vi "HFRR ADV v02.vi"() -> ()   [LabVIEW 2023] (continued)
    n419 = local read "EXIT"() -> (w418:bool)
    "Error Uno" <- w412
  }
  n420 = while {
    tunnel: w47 -> [_]
    tunnel: [w801] -> _
    tunnel: w16 -> [_]
    tunnel: ["EXIT"] -> w44
    i -> [w801]
    stop <- "EXIT" stop-if-true
    # "C:\\LAB-IQ-NXT\\Scar View.exe"
    n421 = local read "RUN"() -> (w799:bool)
    n422 = local read "EDIT 2"() -> (w786:bool)
    n423 = case shown="False" w799 {
      frame False {
        n424 = local read "stopT"() -> (w1691:bool)
        n425 = case shown="True" w1691 {
          frame False {
          }
          frame True {
            w1692 = FALSE
            n426 = local write "st enable"(w1692) -> ()
            n427 = local write "stopT"(w1692) -> ()
          }
        }
      }
      frame True {
        "stopT" <- TRUE
      }
    }
    n428 = case shown="True" w786 {
      frame False {
        n429 = local write "Password 2"("" ("Password")) -> ()
        n430 = property on="Password 2" class="Str"("Visible"=FALSE) -> ()  [unwired: 2 in, 2 out]
      }
      frame True {
        n431 = property on="Password 2" class="Str"("Visible"=TRUE) -> ()  [unwired: 2 in, 2 out]
        n432 = Equal?(x="Password 2", y="HFRR1234") -> (x = y?=w831:bool)
        n433 = case shown="True" w831 {
          tunnel: "Password 2" -> [w834 _]
          frame False {
            n434 = String Length(string=w834) -> (length=w835:i32)
            n435 = Greater Than 0?(x=w835) -> (x > 0?=w833:bool)
            n436 = case shown="False" w833 {
              frame False {
                n437 = property on="Password 2" class="Str"("Caption.Text"="Password (Advance Setting)") -> ()  [unwired: 2 in, 2 out]
              }
              frame True {
                n438 = property on="Password 2" class="Str"("Caption.Text"="Incorrect Password!") -> ()  [unwired: 2 in, 2 out]
              }
            }
          }
          frame True {
            n439 = local write "Password 2"("" ("Password")) -> ()
            n440 = local write "Main Tab"(T1."Advance" ("Main Tab")) -> ()
            n441 = local write "EDIT 2"(FALSE ("EDIT 2")) -> ()
          }
        }
      }
    }
    n442 = Wait (ms)(milliseconds to wait=u32 50) -> ()  [unwired: 1 out]
    n443 = local read "EXIT 2"() -> (w779:bool)
    n444 = local read "Configure"() -> (w782:bool)
    n445 = local read "Analysis"() -> (w781:bool)
    n446 = local read "Home 9"() -> (w776:bool)
    n447 = local read "Home"() -> (w775:bool)
    n448 = local read "STOP 2"() -> (w778:bool)
    n449 = local read "Home 8"() -> (w777:bool)
    n450 = case shown="True" "EDIT 3" {
      frame False {
      }
      frame True {
        n451 = local write "EDIT 3"(FALSE ("EDIT 3")) -> ()
        n452 = local write "Main Tab"(T1."About" ("Main Tab")) -> ()
      }
    }
    n453 = local read "Re-Initialise"() -> (w784:bool)
    n454 = case shown="True" w779 {
      selector: w779 -> [_ w812]
      frame False {
      }
      frame True {
        n455 = local write "EXIT"(w812) -> ()
        n456 = local write "EXIT 2"(FALSE ("EXIT 2")) -> ()
        n457 = local write "Main Tab"(T1."HOME" ("Main Tab")) -> ()
      }
    }
    n458 = case shown="True" w775 {
      frame False {
      }
      frame True {
        (unwired) T10."HOME" ("Main Tab")
        n459 = local write "Home"(FALSE ("Home")) -> ()
        n460 = local write "Main Tab"(T1."HOME" ("Main Tab")) -> ()
      }
    }
    n461 = case shown="True" w784 {
      frame False {
      }
      frame True {
        n462 = local write "Re-Initialise"(FALSE ("Re-Initialise")) -> ()
      }
    }
    n463 = case shown="True" w776 {
      frame False {
      }
      frame True {
        n464 = local write "Main Tab"(T1."HOME" ("Main Tab")) -> ()
        n465 = local write "Home 9"(FALSE ("Home 9")) -> ()
      }
    }
    n466 = case shown="True" w777 {
      frame False {
      }
      frame True {
        n467 = local write "Home 8"(FALSE ("Home 8")) -> ()
        n468 = local write "Main Tab"(T1."HOME" ("Main Tab")) -> ()
      }
    }
    n469 = case shown="True" w778 {
      frame False {
      }
      frame True {
        n470 = local write "STOP 2"(FALSE ("STOP 2")) -> ()
        n471 = local write "Main Tab"(T1."HOME" ("Main Tab")) -> ()
      }
    }
    n472 = case shown="True" w782 {
      frame False {
      }
      frame True {
        n473 = local write "Configure"(FALSE) -> ()
        n474 = local write "Main Tab"(T1."Acquire" ("Main Tab")) -> ()
      }
    }
    n475 = local read "service 2"() -> (w780:bool)
    n476 = case shown="True" w781 {
      frame False {
      }
      frame True {
        n477 = local write "Analysis"(FALSE) -> ()
        n478 = local write "Main Tab"(T1."Compare Files" ("Main Tab")) -> ()
      }
    }
    n479 = case shown="\"ASTM D6079\", Default" "TEST STANDARD" {
      tunnel: [2.0 ("Set Temp") 0.0 ("Set Temp") 2.0 ("Set Temp") 0.0 ("Set Temp")] -> w787
      frame "ASTM D6079", Default {
        # "astm hide"
        n480 = local write "Set Hz"(50.0 ("Hz")) -> ()
        n481 = local write "Set Strk"(1.0 ("Set Strk")) -> ()
        n482 = local write "Set Rh"(53.0 ("Set Rh")) -> ()
        n483 = local write "Set Temp"(60.0 ("Set Temp")) -> ()
        n484 = local write "test time"(75.0 ("test time")) -> ()
        n485 = local write "NORMAL LOAD"(2.0 ("NORMAL LOAD")) -> ()
        "Test Standard" <- "ASTM D6079" ("Test Standard 2")
      }
      frame "ISO 12156" {
        n486 = local write "Set Hz"(50.0 ("Hz")) -> ()
        n487 = local write "Set Rh"(53.0 ("Set Rh")) -> ()
        n488 = local write "Set Strk"(1.0 ("Set Strk")) -> ()
        n489 = local write "test time"(75.0 ("test time")) -> ()
        n490 = local write "Set Temp"(60.0 ("Set Temp")) -> ()
        n491 = local write "NORMAL LOAD"(2.0 ("NORMAL LOAD")) -> ()
      }
      frame "CEC F-096-A-06" {
        n492 = local write "Set Strk"(1.0 ("Set Strk")) -> ()
        n493 = local write "Set Hz"(50.0 ("Hz")) -> ()
        n494 = local write "Set Rh"(53.0 ("Set Rh")) -> ()
        n495 = local write "Set Temp"(60.0 ("Set Temp")) -> ()
        n496 = local write "test time"(75.0 ("test time")) -> ()
        n497 = local write "NORMAL LOAD"(2.0 ("NORMAL LOAD")) -> ()
      }
      frame "Custom" {
      }
    }
    n498 = local read "OPEN 6"() -> (w783:bool)
    n499 = local read "service 3"() -> (w773:bool)
    n500 = case shown="True" w780 {
      frame False {
      }
      frame True {
        n501 = local write "service 2"(FALSE) -> ()
        n502 = local write "Main Tab"(T1."About" ("Main Tab")) -> ()
      }
    }
    n503 = Or(x=w783, y=w773) -> (x .or. y?=w774:bool)
    n504 = local read "RUN"() -> (w796:bool)
    n505 = case shown="True" w774 {
      selector: w774 -> [_ w823]
      frame False {
      }
      frame True {
        n506 = Not(x=w823) -> (.not. x?=w819:bool)
        n507 = local write "service 3"(w819) -> ()
        n508 = local write "OPEN 6"(w819) -> ()
        n509 = call <vilib>:"System Exec.vi"("wait until completion? (T)"=TRUE, "command line"="C:\\LAB-IQ-NXT\\Scar View.exe") -> ("error out"=→"error out 5":errorcluster)  [unwired: 6 in, 3 out]
      }
    }
    n510 = case shown="True" w796 {
      frame False {
      }
      frame True {
        n511 = local read "Main Tab"() -> (w1689:T1)
        n512 = case shown="\"Compare Files\"" w1689 {
          frame "Acquire", Default {
          }
          frame "Compare Files" {
            n513 = local write "Main Tab"(T1."Acquire" ("Main Tab")) -> ()
          }
          frame "About" {
          }
        }
      }
    }
    n514 = local read "Main Tab"() -> (w772:T1)
    n515 = case shown="\"Compare Files\"" w772 {
      tunnel: [T10."Acquire" ("Main Tab") T11."   COMPARE   FILES " ("Tab Control") T12."PRINT REPORT" ("Tab Control")] -> w794
      frame "Acquire", Default {
      }
      frame "Compare Files" {
      }
      frame "About" {
      }
    }
    n516 = property on="SetTemp" class="DigNum (strict)"("Disabled"=w787) -> ()  [unwired: 2 in, 2 out]
    n517 = case shown="0, Default" w794 {
      frame 0, Default {
        w1833 = 0.2 ("y")
        w1838 = 1.0 ("y")
        w1839 = 0.8 ("y")
        # "Elapsed time\ncof\nstroke\nAir temp\nTemp\nHumidity"
        n518 = case shown="True" "Save & Continue" {
          frame False {
          }
          frame True {
            "acq 2" <- TRUE ("acq 2")
          }
        }
        n519 = case shown="True" "Save & Continue" {
          frame False {
          }
          frame True {
            n520 = while {
              tunnel: "0123456789abcdefghijklmnopqrstuvwxyzABCDEFGHIJKLMNOPQRSTUVWXYZ" ("string 2") -> [w1957]
              shift-right: [w1955] -> w1950
              shift-left: "" -> [w1954]
              i -> [w1964]
              stop <- w1963 stop-if-true
              n521 = Random Number (0-1)() -> (number: 0 to 1=w1958:dbl)
              n522 = Multiply(x=w1958, y=62.0) -> (x*y=w1960:dbl)
              n523 = Decrement(x="Length") -> (x-1=w1953:i16)
              n524 = To Word Integer(number=w1960) -> (16bit integer=w1961:i16)
              n525 = String Subset(string=w1957, offset (0)=w1961, length (rest)=1 ("length (rest)")) -> (substring=w1956:string)
              n526 = Greater Or Equal?(x=w1964, y=w1953) -> (x >= y?=w1963:bool)
              n527 = Concatenate Strings(w1956, w1954) -> (w1955:string)
            }
            n528 = local write "UUID"(w1950) -> ()
          }
        }
        n529 = case shown="True" "Save & Continue" {
          frame False {
          }
          frame True {
            n530 = local read "Operator ID"() -> (w2240:string)
            n531 = local read "FILE"() -> (w2247:string)
            n532 = String Length(string=w2240) -> (length=w2241:i32)
            n533 = String Length(string=w2247) -> (length=w2245:i32)
            n534 = Greater?(x=w2241, y=0) -> (0:w2239:bool)
            n535 = Greater?(x=w2245, y=0) -> (0:w2244:bool)
            n536 = And(x=w2244, y=w2239) -> (x .and. y?=w2243:bool)
            n537 = case shown="True" w2243 {
              frame False {
                n538 = stacked-sequence {
                  frame #0 {
                    n539 = One Button Dialog(message="Please Enter a File Name and Operator ID to save data !", button name ("OK")="Ok") -> ()  [unwired: 1 out]
                  }
                  frame #1 {
                    n540 = local write "Save & Continue"(FALSE ("OK Button")) -> ()
                  }
                }
                n541 = local write "Save & Continue"(FALSE ("OK Button")) -> ()
              }
              frame True {
                n542 = stacked-sequence {
                  frame #0 {
                    (unwired) ")!" ("string")
                    (unwired) ")" ("string")
                    w2252 = dbl[] [] ("History Data")
                    w2256 = "\r"
                    # "C:\\WinDucom\\Data\\"
                    # "C:\\LAB-IQ-NXT\\data"
                    n543 = local read "Batch Ref Num :"() -> (w2254:string)
                    n544 = local read "NORMAL LOAD"() -> (w2273:dbl)
                    n545 = local read "Fuel Discription :"() -> (w2267:string)
                    n546 = Multiply(x=w2273, y=1.0) -> (x*y=w2272:dbl)
                    n547 = Number To Fractional String(number=w2272, width (-)=i16 5, precision (6)=i16 2) -> (F-format string=w2281:string)  [unwired: 1 in]
                    n548 = Concatenate Strings(w2267) -> (w2268:string)
                    n549 = local read "Remarks :"() -> (w2266:string)
                    n550 = property on="Electronic contact resistance ( % )" class="WFChart (strict)"("History Data"=w2252) -> ()  [unwired: 2 in, 2 out]
                    n551 = Get Date/Time String(date format (0)=enum16{"short", "long", "abbreviated"}."short") -> (date string=w2292:string, time string=w2289:string)  [unwired: 2 in]
                    n552 = property on="Coefficient of Friction" class="WFChart (strict)"("History Data"=w2252) -> ()  [unwired: 2 in, 2 out]
                    n553 = property on="Frictional Force ( N )" class="WFChart (strict)"("History Data"=w2252) -> ()  [unwired: 2 in, 2 out]
                    n554 = Concatenate Strings(w2254) -> (w2253:string)
                    n555 = Concatenate Strings(w2266, "," ("string")) -> (w2265:string)
                    n556 = Concatenate Strings("Load :- " ("Substring"), w2281, " N ," ("Substring")) -> (w2280:string)
                    n557 = local read "String 41"() -> (w2258:string)
                    n558 = local read "FILE"() -> (w2300:string)
                    n559 = Concatenate Strings("(" ("Substring"), w2292, ")" ("Substring"), w2289) -> (w2260:string)
                    "concatenated string" <- w2260
                    n560 = Concatenate Strings("C:\\LAB-IQ-NXT\\data\\" ("string"), w2300) -> (w2299:string)
                    n561 = Concatenate Strings("tested by") -> (w2262:string)
                    n562 = Concatenate Strings(w2299, ".duf" ("Substring")) -> (w2296:string)
                    n563 = Concatenate Strings(w2299, ".dgf" ("Substring")) -> (w2295:string)
                    n564 = String To Path(string=w2295) -> (path=w2293:path)
                    n565 = String To Path(string=w2296) -> (path=w2270:path)
                    n566 = Concatenate Strings(w2258, w2256, "Fuel Discription :-" ("Substring"), w2268, w2256, w2280, w2256, "Batch Ref Num :-" ("Substring"), w2253, w2256, " Remarks :- " ("Substring"), w2265, w2256, " Date :- " ("Substring"), w2260, w2256, "Tested By :-" ("Substring"), w2262) -> (w2274:string)
                    "REMARKS" <- w2274
                    n567 = local write "clk"(0.0 ("clk")) -> ()
                    n568 = local write "speedop"(0.0 ("PIDclk 2")) -> ()
                    n569 = Concatenate Strings("  TIME;      COF;       STROKE;     AIR TEMP;  TEMP;  HUMIDITY;  ECR; PID-OUT; FREQUENCY" ("Substring"), "\r") -> (w2276:string)
                    n570 = call <vilib>:"Write Characters To File.vi"("append to file? (new file:F)"=FALSE, "character string"=w2276, "file path (dialog if empty)"=w2293) -> ()  [unwired: 2 in, 1 out]
                    n571 = call <vilib>:"Write Characters To File.vi"("append to file? (new file:F)"=FALSE, "character string"=w2274, "file path (dialog if empty)"=w2270) -> ()  [unwired: 2 in, 1 out]
                  }
                  frame #1 {
                    n572 = local write "autostrtflg"(TRUE ("autostrtflg")) -> ()
                    n573 = local write "Save & Continue"(FALSE ("OK")) -> ()
                    n574 = local write "STOP 3"(FALSE ("STOP")) -> ()
                    n575 = One Button Dialog(message="Please ensure sample is mounted properly and machine is ready in all aspects for testing !", button name ("OK")="Ok") -> ()  [unwired: 1 out]
                    n576 = property on="Save & Continue" class="Bool (strict)"("Visible"=FALSE ("OK")) -> ()  [unwired: 2 in, 2 out]
                    n577 = property on="STOP 3" class="Bool (strict)"("Visible"=TRUE) -> ()  [unwired: 2 in, 2 out]
                    n578 = Get Date/Time In Seconds() -> (seconds since 1Jan1904=w2305:timestamp)
                    n579 = local write "Cycles elapsed"(0 ("Cycles elapsed")) -> ()
                    n580 = To Double Precision Float(number=w2305) -> (double precision float=w2304:dbl)
                    n581 = local write "cyclecount"(0 ("cyclecount")) -> ()
                    n582 = local write "acq timer"(w2304) -> ()
                    n583 = local write "Save"(FALSE ("Save")) -> ()
                  }
                }
              }
            }
          }
        }
        n584 = case shown="True" "Case Constant\n(See Context Help) 15" {
          frame False {
          }
          frame True {
            n585 = local read "zflag 2"() -> (w1865:dbl)
            n586 = local read "yflag"() -> (w1867:dbl)
            n587 = Equal?(x=w1865, y=3.0 ("tflag")) -> (x = y?=w1868:bool)
            n588 = Equal?(x=w1867, y=2.0 ("tflag")) -> (x = y?=w1869:bool)
            n589 = And(x=w1869, y=w1868) -> (x .and. y?=w1863:bool)
            n590 = case shown="True" w1863 {
              frame False {
              }
              frame True {
                w1894 = 0.0 ("zflag")
                n591 = local read "SEN.RUN HRS"() -> (w1880:dbl)
                n592 = local read "SENSOR TIME"() -> (w1878:dbl)
                n593 = local read "Total No. of Tests"() -> (w1881:dbl)
                n594 = Delete(path (use dialog)=path "C:/LAB-IQ-NXT/WO 2449 TRH.sig" ("file path (dialog if empty)")) -> (deleted path=w1888:path)  [unwired: 4 in, 2 out]
                n595 = Add(x=w1878, y=w1880) -> (x+y=w1879:dbl)
                "SEN.RUN HRS" <- w1879
                n596 = Number To Decimal String(number=w1879) -> (decimal integer string=w1885:string)  [unwired: 1 in]
                n597 = call <vilib>:"compatOverwrite.vi"("overwrite (F)"=TRUE) -> ("overwrite?"=w1874:T15)
                n598 = Delete(path (use dialog)=path "C:/LAB-IQ-NXT/WO 2449 TT.sig" ("file path (dialog if empty)")) -> (deleted path=w1893:path)  [unwired: 4 in, 2 out]
                n599 = Open/Create/Replace File(file path (use dialog)=w1888, operation (0:open)=w1874) -> (refnum out=w1875:refnum<file>, error out=w1876:errorcluster)  [unwired: 4 in, 1 out]
                n600 = Number To Decimal String(number=w1881) -> (decimal integer string=w1889:string)  [unwired: 1 in]
                n601 = Deny Access(4:w1876, 6:T13."deny none" ("deny mode (2)"), 7:w1875) -> (3:w1884:refnum<file>)  [unwired: 1 out]
                n602 = call <vilib>:"compatOverwrite.vi"("overwrite (F)"=TRUE) -> ("overwrite?"=w1870:T15)
                n603 = Write to Binary File(file (use dialog)=w1884, data=w1885, 5:FALSE ("prepend array or string size? (T)")) -> ()  [unwired: 3 in, 3 out]
                n604 = Open/Create/Replace File(file path (use dialog)=w1893, operation (0:open)=w1870) -> (refnum out=w1871:refnum<file>, error out=w1872:errorcluster)  [unwired: 4 in, 1 out]
                n605 = Deny Access(4:w1872, 6:T13."deny none" ("deny mode (2)"), 7:w1871) -> (3:w1892:refnum<file>)  [unwired: 1 out]
                n606 = local write "zflag"(w1894) -> ()
                n607 = local write "zflag 2"(w1894) -> ()
                n608 = Write to Binary File(file (use dialog)=w1892, data=w1889, 5:FALSE ("prepend array or string size? (T)")) -> ()  [unwired: 3 in, 3 out]
              }
            }
          }
        }
        n609 = case shown="True" "STOP 3" {
          frame False {
          }
          frame True {
            w2232 = "" ("Sample ID :")
            (unwired) FALSE ("Visible")
            n610 = local write "Save & Continue"(FALSE ("OK Button")) -> ()
            n611 = local write "STOP 3"(FALSE ("STOP")) -> ()
            n612 = local write "clk"(0.0 ("clk")) -> ()
            n613 = local write "RUN"(FALSE ("OK Button 2")) -> ()
            n614 = property on="Save & Continue" class="Bool (strict)"("Visible"=TRUE) -> ()  [unwired: 2 in, 2 out]
            n615 = property on="STOP 3" class="Bool (strict)"("Visible"=FALSE) -> ()  [unwired: 2 in, 2 out]
            n616 = property on="STOP 2" class="Bool (strict)"("Disabled"=u8 0) -> ()  [unwired: 2 in, 2 out]
            n617 = local write "Fuel Discription :"(w2232) -> ()
            n618 = local write "Remarks :"(w2232) -> ()
            n619 = local write "tested by"(w2232) -> ()
            n620 = local write "FILE"(w2232) -> ()
            n621 = local write "Batch Ref Num :"(w2232) -> ()
          }
        }
        n622 = local read "AIR TEMP"() -> (w1805:dbl)
        n623 = local read "run replace"() -> (w1845:bool)
        n624 = Greater Or Equal?(x=w1805, y=15.0) -> (x >= y?=w1806:bool)
        "powstat" <- w1806
        n625 = local read "acq 2"() -> (w1844:bool)
        n626 = And(x=w1844, y=w1845) -> (x .and. y?=w1843:bool)
        n627 = local read "run replace"() -> (w1846:bool)
        n628 = case shown="True" w1843 {
          frame False {
            n629 = local write "tfalg"(0.0 ("tfalg")) -> ()
          }
          frame True {
            n630 = local read "tfalg"() -> (w1941:dbl)
            n631 = Equal?(x=w1941, y=0.0) -> (x = y?=w1942:bool)
            n632 = case shown="True" w1942 {
              frame False {
              }
              frame True {
                n633 = local read "Total No. of Tests"() -> (w1945:dbl)
                n634 = Increment(x=w1945) -> (x+1=w1944:dbl)
                n635 = local write "Total No. of Tests"(w1944) -> ()
                n636 = local write "tfalg"(1.0 ("tfalg")) -> ()
                n637 = local write "acq 2"(FALSE ("acq 2")) -> ()
                n638 = Wait (ms)(milliseconds to wait=u32 200) -> ()  [unwired: 1 out]
              }
            }
          }
        }
        n639 = case shown="False" w1846 {
          frame False {
            n640 = local read "zflag"() -> (→"zflag 2":dbl)
            n641 = local write "FLAG 4"(0.0 ("FLAG")) -> ()
            n642 = local write "yflag"(2.0 ("tflag")) -> ()
          }
          frame True {
            n643 = local write "zflag"(3.0 ("zflag")) -> ()
            n644 = local write "yflag"(1.0 ("tflag")) -> ()
          }
        }
        n645 = property on="STOP 3" class="Bool (strict)"() -> ("Visible"=w1848:bool)  [unwired: 2 in, 2 out]
        n646 = case shown="True" w1848 {
          tunnel: [FALSE ("Visible") TRUE ("Visible")] -> w1858
          frame False {
          }
          frame True {
          }
        }
        n647 = property on="RUN" class="Bool (strict)"("Visible"=w1858) -> ()  [unwired: 2 in, 2 out]
        n648 = property on="Save & Continue" class="Bool (strict)"() -> ("Visible"=w1861:bool)  [unwired: 2 in, 2 out]
        n649 = local read "RUN"() -> (w1842:bool)
        n650 = case shown="True" w1842 {
          frame False {
            n651 = local read "Rt 3"() -> (w1923:bool)
            n652 = case shown="True" w1923 {
              frame False {
              }
              frame True {
                n653 = local write "Json End Flg"(TRUE ("Upld AR 2")) -> ()
                n654 = local write "Rt 3"(FALSE ("Rt 3")) -> ()
              }
            }
            "Rt" <- TRUE ("Rt")
            "Rt 2" <- FALSE ("Rt")
          }
          frame True {
            n655 = local read "Rt"() -> (w1930:bool)
            n656 = case shown="True" w1930 {
              frame False {
              }
              frame True {
                w1931 = TRUE ("Upld AR 2")
                n657 = local write "Rt"(FALSE ("Rt")) -> ()
                n658 = local write "Upld AR"(w1931) -> ()
                n659 = local write "Json St Flg"(w1931) -> ()
              }
            }
            n660 = local write "Rt 2"(TRUE ("Rt 2")) -> ()
            "Rt 3" <- TRUE ("Rt 3")
          }
        }
        n661 = Not(x=w1861) -> (.not. x?=w1860:bool)
        n662 = case shown="True" w1842 {
          frame False {
            n663 = local write "run replace"(FALSE ("run replace")) -> ()
          }
          frame True {
            "run replace" <- TRUE ("run replace")
          }
        }
        n664 = And(x=w1860, y=w1848) -> (x .and. y?=w1857:bool)
        "Test Status 2" <- w1857
        n665 = case shown="True" w1857 {
          tunnel: w1806 -> [_ w1996]
          frame False {
            w1994 = 0.0 ("output")
            n666 = local write "Frequency ( Hz )"(w1994) -> ()
            n667 = local write "PID-out"(w1994) -> ()
            n668 = local write "Heater Button"(FALSE ("Heater Button")) -> ()
          }
          frame True {
            n669 = case shown="False" w1996 {
              frame False {
                n670 = stacked-sequence {
                  frame #0 {
                    n671 = local write "RUN"(FALSE ("OK Button 2")) -> ()
                  }
                  frame #1 {
                    n672 = property on="RUN" class="Bool (strict)"("Visible"=FALSE) -> ()  [unwired: 2 in, 2 out]
                  }
                }
              }
              frame True {
              }
            }
            n673 = stacked-sequence {
              frame #0 {
                n674 = case shown="True" "RUN" {
                  tunnel: [w2023 w2031] -> w2000
                  frame False {
                    w2023 = 0.0
                    n675 = local write "Reinit PID"(TRUE) -> ()
                    n676 = property on="Stroke 2" class="DigNum (strict)"("Visible"=FALSE) -> ()  [unwired: 2 in, 2 out]
                    n677 = property on="Stroke" class="DigNum (strict)"("Visible"=TRUE) -> ()  [unwired: 2 in, 2 out]
                    n678 = local write "String 14"("Test will autostart once parameters reach the set value." ("String 14")) -> ()
                    n679 = local write "Old Pid Val"(w2023) -> ()
                  }
                  frame True {
                    n680 = local read "PID Ref"() -> (w2042:bool)
                    n681 = property on="STOP 2" class="Bool (strict)"("Disabled"=u8 2) -> ()  [unwired: 2 in, 2 out]
                    n682 = case shown="True" w2042 {
                      tunnel: [w2043 w2059] -> w2041
                      frame False {
                        n683 = local read "Old Pid Val"() -> (w2043:dbl)
                      }
                      frame True {
                        n684 = local read "Set Hz"() -> (w2052:dbl)
                        n685 = Add(x=w2052, y=-10.0 ("Offset")) -> (x+y=w2070:dbl)
                        n686 = local read "Frequency"() -> (w2063:dbl)
                        n687 = Add(x=w2052, y=-10.0) -> (x+y=w2062:dbl)
                        n688 = Add(x=w2052, y=10.0) -> (x+y=w2061:dbl)
                        n689 = Multiply(x=w2070, y=0.1 ("Gain")) -> (x*y=w2049:dbl)
                        n690 = Add(x=w2049, y=1.5) -> (x+y=w2047:dbl)
                        n691 = local read "SPEED OUT:"() -> (w2071:dbl)
                        n692 = In Range and Coerce(upper limit=w2061, x=w2063, lower limit=w2062) -> (coerced(x)=w2051:dbl)  [unwired: 1 out]
                        n693 = Multiply(x=w2047, y=w2071) -> (x*y=w2046:dbl)
                        n694 = Multiply(x=w2046, y=0.8) -> (x*y=w2045:dbl)
                        n695 = local read "Elapsed time"() -> (w2056:dbl)
                        n696 = Or(x="Reinit PID", y="Reinit PID") -> (x .or. y?=w2060:bool)
                        n697 = call-poly <vilib>:"PID.vi"("reinitialize? (F)"=w2060, "output range"=cluster{"output high":dbl, "output low":dbl} {"output high"=1.0, "output low"=-1.0}, "PID gains"=T7 {"proportional gain (Kc)"=0.0005, "integral time (Ti, min)"=0.001, "derivative time (Td, min)"=0.0} ("Motor PID"), "process variable"=w2051, "setpoint"=w2052) -> ("output"=w2050:dbl)  [unwired: 5 in, 1 out]
                        n698 = Greater?(x=w2056, y=0.05) -> (0:w2055:bool)
                        n699 = case shown="True" w2055 {
                          tunnel: w2050 -> [_ w2073]
                          tunnel: [0.0 ("output") w2073] -> w2053
                          frame False {
                          }
                          frame True {
                            n700 = local write "Reinit PID"(FALSE ("Reinit PID")) -> ()
                          }
                        }
                        n701 = Add(x=w2045, y=w2053) -> (x+y=w2058:dbl)
                        n702 = flat-sequence {
                          tunnel: [w2076] -> w2059
                          tunnel: w2058 -> [w2076]
                          frame #0 {
                            n703 = local write "PID Ref"(FALSE ("PID Ref")) -> ()
                          }
                        }
                      }
                    }
                    "Old Pid Val" <- w2041
                    n704 = local read "Set Hz"() -> (w2038:dbl)
                    n705 = local read "Freq"() -> (w2030:dbl)
                    n706 = call <vilib>:"Uniform White Noise Waveform.vi"() -> ("signal out"=w2037:waveform(dbl))  [unwired: 10 in, 1 out]
                    n707 = property on="RUN" class="Bool (strict)"("Visible"=TRUE) -> ()  [unwired: 2 in, 2 out]
                    n708 = Add(x=w2038, y=w2037) -> (x+y=w2036:waveform(dbl))
                    n709 = property on="Stroke 2" class="DigNum (strict)"("Visible"=TRUE) -> ()  [unwired: 2 in, 2 out]
                    n710 = property on="Stroke" class="DigNum (strict)"("Visible"=FALSE) -> ()  [unwired: 2 in, 2 out]
                    n711 = Multiply(x=w2036, y=ext 0.1) -> (x*y=w2032:waveform(ext))
                    n712 = Multiply(x=w2030, y=0.9) -> (x*y=w2033:dbl)
                    n713 = local write "String 14"(" Running....." ("String 14")) -> ()
                    n714 = Add(x=w2032, y=w2033) -> (x+y=w2031:waveform(ext))
                  }
                }
                n715 = Not(x="Engage") -> (.not. x?=w2004:bool)
                n716 = call "Elapsed Time"("Time Target (s)"="Countdown", "Reset"=w2004) -> ("Elapsed Time (s)"=w2009:dbl, "Time has Elapsed"=w2007:bool)  [unwired: 10 in, 6 out]
                "Countdown 2" <- w2009
                n717 = Subtract(x=w2009, y=2.0) -> (x-y=w2012:dbl)
                n718 = Less?(x=w2012, y="Countdown") -> (x < y?=w2010:bool)
                n719 = And(x=w2010, y=w2007) -> (x .and. y?=w2006:bool)
                n720 = case shown="True" w2006 {
                  frame False {
                  }
                  frame True {
                    n721 = local read "Humidity ( Rh )"() -> (→"Rh Before":dbl)
                    n722 = local write "RUN"(TRUE ("RUN")) -> ()
                    n723 = local write "Engage"(FALSE ("Engage")) -> ()
                    n724 = property on="gRh" class="WFChart (strict)"("History Data"=dbl[] []) -> ()  [unwired: 2 in, 2 out]
                  }
                }
                n725 = local read "clk"() -> (w2017:dbl)
                n726 = local read "Save"() -> (w2013:bool)
                n727 = Equal?(x=w2017, y=0.0) -> (x = y?=w2014:bool)
                n728 = And(x=w2014, y=w2013) -> (x .and. y?=w2015:bool)
                n729 = case shown="True" w2015 {
                  frame False {
                  }
                  frame True {
                    n730 = Get Date/Time In Seconds() -> (seconds since 1Jan1904=w2079:timestamp)
                    n731 = To Double Precision Float(number=w2079) -> (double precision float=w2077:dbl)
                    n732 = local write "act save time"(w2077) -> ()
                    n733 = local write "acq timer"(w2077) -> ()
                    n734 = local write "clk"(10.0 ("clk")) -> ()
                  }
                }
                n735 = local read "Test \nStatus"() -> (w2002:bool)
                n736 = Select(t=w2000, s=w2002, f=0.0) -> (s? t:f=w2001:dbl)
                n737 = local write "Frequency ( Hz )"(w2001) -> ()
                n738 = local write "Freq"(w2001) -> ()
              }
              frame #1 {
                w2102 = 1000000.0 ("x")
                # "Elapsed time\ncof\nstroke\nAir temp\nTemp\nHumidity"
                # "acq timer\n\nact save time"
                # "convert to microseconds"
                n739 = local read "COUNT"() -> (w2085:i32)
                n740 = Greater Or Equal?(x=w2085, y=250) -> (x >= y?=w2084:bool)
                n741 = case shown="True" w2084 {
                  frame False {
                    n742 = local read "COUNT"() -> (w2106:i32)
                    n743 = Increment(x=w2106) -> (x+1=w2107:i32)
                    n744 = local write "COUNT"(w2107) -> ()
                  }
                  frame True {
                    n745 = local write "COUNT"(0 ("COUNT")) -> ()
                  }
                }
                n746 = local read "Samplingtime 2"() -> (w2083:dbl)
                n747 = local read "act save time"() -> (w2100:dbl)
                n748 = Get Date/Time In Seconds() -> (seconds since 1Jan1904=w2105:timestamp)
                n749 = To Double Precision Float(number=w2105) -> (double precision float=w2094:dbl)
                n750 = local read "acq timer"() -> (w2104:dbl)
                n751 = Add(x=w2100, y=w2083) -> (x+y=w2099:dbl)
                n752 = Greater Or Equal?(x=w2094, y=w2099) -> (x >= y?=w2082:bool)
                n753 = Subtract(x=w2094, y=w2104) -> (x-y=w2096:dbl)
                n754 = local read "Rate"() -> (w2098:dbl)
                n755 = Divide(x=w2102, y=w2098) -> (x/y=w2103:dbl)
                n756 = Divide(x=w2103, y=w2102) -> (x/y=w2101:dbl)
                n757 = local read "Save"() -> (w2097:bool)
                n758 = And(x=w2082, y=w2097) -> (x .and. y?=w2095:bool)
                n759 = case shown="True" w2095 {
                  tunnel: w2094 -> [_ w2177]
                  tunnel: [FALSE ("Boolean 2") TRUE ("Boolean 2")] -> _
                  frame False {
                  }
                  frame True {
                    w2145 = ";" ("Substring")
                    # "Pid out/\nFreq response value"
                    n760 = local write "act save time"(w2177) -> ()
                    n761 = local read "Set Strk"() -> (w2144:dbl)
                    n762 = local read "Stroke"() -> (w2134:dbl)
                    n763 = local read "FF 2"() -> (w2130:dbl)
                    "Frictional Force ( N )" <- w2130
                    n764 = Subtract(x=w2134, y=w2144) -> (x-y=w2141:dbl)
                    n765 = local read "TEMP"() -> (w2131:dbl)
                    "Temp" <- w2131
                    n766 = local write "FF 3"(w2130) -> ()
                    n767 = local read "ecr"() -> (w2129:dbl)
                    "ecr 2" <- w2129
                    n768 = Multiply(x=w2141, y=0.05) -> (x*y=w2143:dbl)
                    n769 = local read "Humidity ( Rh )"() -> (w2152:dbl)
                    "gRh" <- w2152
                    n770 = local read "Frequency ( Hz )"() -> (w2137:dbl)
                    n771 = local write "ecr 3"(w2129) -> ()
                    n772 = local read "COF 2"() -> (w2132:dbl)
                    "cof" <- w2132
                    "Coefficient of Friction" <- w2132
                    n773 = Add(x=w2143, y=w2144) -> (x+y=w2135:dbl)
                    "Stroke Ln" <- w2135
                    "Stroke 2" <- w2135
                    "Disp" <- w2135
                    n774 = local write "Temperature ( Deg C )"(w2131) -> ()
                    n775 = local read "Elapsed time"() -> (w2170:dbl)
                    n776 = local write "COF 3"(w2132) -> ()
                    n777 = local read "AIR TEMP"() -> (w2133:dbl)
                    n778 = local write "Electronic contact resistance ( % )"(w2129) -> ()
                    n779 = local read "PID-out"() -> (w2140:dbl)
                    n780 = local read "FILE"() -> (w2178:string)
                    n781 = Number To Fractional String(number=w2132, width (-)=i16 9 ("precision (6)"), precision (6)=i16 6) -> (F-format string=w2171:string)  [unwired: 1 in]
                    n782 = Number To Fractional String(number=w2135, width (-)=i16 9 ("precision (6)"), precision (6)=i16 6) -> (F-format string=w2163:string)  [unwired: 1 in]
                    n783 = Number To Fractional String(number=w2133, width (-)=i16 9 ("precision (6)"), precision (6)=i16 3) -> (F-format string=w2162:string)  [unwired: 1 in]
                    n784 = Number To Fractional String(number=w2131, width (-)=i16 9 ("precision (6)"), precision (6)=i16 3) -> (F-format string=w2159:string)  [unwired: 1 in]
                    n785 = Number To Fractional String(number=w2152, width (-)=i16 9 ("precision (6)"), precision (6)=i16 3) -> (F-format string=w2156:string)  [unwired: 1 in]
                    n786 = Number To Fractional String(number=w2129, width (-)=i16 9 ("precision (6)"), precision (6)=i16 3) -> (F-format string=w2151:string)  [unwired: 1 in]
                    n787 = Number To Fractional String(number=w2140, width (-)=i16 9 ("precision (6)"), precision (6)=i16 3) -> (F-format string=w2146:string)  [unwired: 1 in]
                    n788 = Number To Fractional String(number=w2137, width (-)=i16 9 ("precision (6)"), precision (6)=i16 3) -> (F-format string=w2136:string)  [unwired: 1 in]
                    n789 = Number To Fractional String(number=w2170, width (-)=i16 14 ("precision (6)"), precision (6)=i16 3) -> (F-format string=w2172:string)  [unwired: 1 in]
                    n790 = Concatenate Strings("C:\\LAB-IQ-NXT\\Data\\" ("string"), w2178, ".dgf" ("Substring")) -> (w2180:string)
                    n791 = String To Path(string=w2180) -> (path=w2179:path)
                    n792 = Concatenate Strings(w2172, w2145, w2171, w2145, w2163, w2145, w2162, w2145, w2159, w2145, w2156, w2145, w2151, w2145, w2146, w2145, w2136, "\r") -> (w2169:string)
                    n793 = call <vilib>:"Write Characters To File.vi"("append to file? (new file:F)"=TRUE, "character string"=w2169, "file path (dialog if empty)"=w2179) -> ()  [unwired: 2 in, 1 out]
                    "refresh flag" <- TRUE ("refresh flag")
                  }
                }
                n794 = local read "COUNT"() -> (w2087:i32)
                n795 = Multiply(x=w2101, y=w2087) -> (x*y=w2093:dbl)
                n796 = Add(x=w2096, y=w2093) -> (x+y=w2080:dbl)
                "Elapsed time 3" <- w2080
                n797 = local read "Test \nStatus"() -> (w2081:bool)
                n798 = local read "clk"() -> (w2088:dbl)
                n799 = Equal?(x=w2088, y=10.0) -> (x = y?=w2090:bool)
                n800 = Divide(x=w2080, y=60.0) -> (x/y=w2091:dbl)
                n801 = case shown="True" w2081 {
                  tunnel: w2091 -> [_ w2113]
                  tunnel: w2096 -> [_ w2121]
                  tunnel: [0.0 w2117] -> _
                  tunnel: w2090 -> [_ w2116]
                  tunnel: [0.0 w2115] -> _
                  tunnel: w2080 -> [_ w2115]
                  tunnel: w2094 -> [w2109 _]
                  frame False {
                    n802 = local write "acq timer"(w2109) -> ()
                  }
                  frame True {
                    n803 = local read "Set Hz"() -> (w2118:dbl)
                    n804 = local write "Elapsed time"(w2113) -> ()
                    n805 = local read "test time"() -> (w2114:dbl)
                    n806 = Multiply(x=w2121, y=w2118) -> (x*y=w2120:dbl)
                    n807 = case shown="False" w2116 {
                      tunnel: w2120 -> [w2122 _]
                      tunnel: [w2122 1.0] -> w2117
                      frame False {
                        n808 = local write "Cycles elapsed"(w2122) -> ()
                      }
                      frame True {
                      }
                    }
                    n809 = Subtract(x=w2114, y=w2113) -> (x-y=w2112:dbl)
                    "time" <- w2112
                    n810 = Greater?(x=w2113, y=w2114) -> (0:w2119:bool)
                    n811 = case shown="True" w2119 {
                      frame False {
                      }
                      frame True {
                        n812 = local read "Humidity ( Rh )"() -> (→"Rh After":dbl)
                        n813 = property on="STOP 2" class="Bool (strict)"("Disabled"=u8 0) -> ()  [unwired: 2 in, 2 out]
                        n814 = local write "RUN"(FALSE ("OK Button 2")) -> ()
                        n815 = local write "STOP 3"(TRUE ("STOP")) -> ()
                      }
                    }
                    n816 = local write "Time Remaining"(w2112) -> ()
                  }
                }
              }
              frame #2 {
                n817 = case shown="True" "Heater Button" {
                  tunnel: [0.0 ("output") w2204] -> w2183
                  frame False {
                    w2185 = TRUE ("tmpchk")
                    n818 = local write "tmpchk"(w2185) -> ()
                    n819 = local write "Reset 4"(w2185) -> ()
                    n820 = local read "TEMP"() -> (w2186:dbl)
                    n821 = local write "Temp ini"(w2186) -> ()
                    n822 = local write "reinit"(TRUE ("reinit")) -> ()
                  }
                  frame True {
                    # "Logic to turn off\nthe heater when \ntemp is not rising.\nTime - 60 sec\nDelta t- 5°c"
                    n823 = local read "Set Temp"() -> (w2201:dbl)
                    n824 = local read "Temp ini"() -> (w2192:dbl)
                    n825 = local read "TEMP"() -> (w2195:dbl)
                    n826 = Add(x=w2201, y=0.5) -> (x+y=w2199:dbl)
                    n827 = Less?(x=w2192, y=53.0) -> (x < y?=w2190:bool)
                    n828 = Greater Or Equal?(x=w2195, y=w2199) -> ()  [unwired: 1 out]
                    n829 = And(x="tmpchk", y=w2190) -> (x .and. y?=w2193:bool)
                    n830 = case shown="True" w2193 {
                      frame False {
                      }
                      frame True {
                        n831 = call "Elapsed Time8"("Time Target (s)"=300.0, "Reset"="Reset 4") -> ("Time has Elapsed"=w2209:bool)  [unwired: 10 in, 7 out]
                        n832 = flat-sequence {
                          tunnel: w2209 -> [_]
                          frame #0 {
                            n833 = local write "Reset 4"(FALSE ("Reset 4")) -> ()
                          }
                        }
                        n834 = case shown="True" w2209 {
                          frame False {
                          }
                          frame True {
                            n835 = local read "Temp ini"() -> (w2216:dbl)
                            n836 = local read "TEMP"() -> (w2217:dbl)
                            n837 = Add(x=w2216, y=5.0) -> (x+y=w2214:dbl)
                            n838 = Greater?(x=w2217, y=w2214) -> (0:w2215:bool)
                            n839 = case shown="False" w2215 {
                              frame False {
                                n840 = local write "Heater Button"(FALSE ("Heater Button")) -> ()
                              }
                              frame True {
                                n841 = local write "tmpchk"(FALSE ("tmpchk")) -> ()
                              }
                            }
                          }
                        }
                      }
                    }
                    n842 = call-poly <vilib>:"PID.vi"("reinitialize? (F)"="reinit", "output range"="output range", "dt (s)"=-1.0, "PID gains"="Temp PID gains", "process variable"=w2195, "setpoint"=w2201) -> ("output"=w2198:dbl)  [unwired: 4 in, 1 out]
                    n843 = Select(t=0.0, s=FALSE, f=w2198) -> (s? t:f=w2197:dbl)
                    "PID output" <- w2197
                    n844 = Subtract(x=w2201, y=w2195) -> (x-y=w2203:dbl)
                    n845 = flat-sequence {
                      tunnel: w2197 -> [w2220]
                      tunnel: [w2220] -> w2204
                      frame #0 {
                        n846 = local write "reinit"(FALSE ("reinit")) -> ()
                      }
                    }
                    n847 = Bundle(w2203, "output"=w2197, "TEMP"=w2195) -> (→"gTEMP 3":cluster{dbl, "output":dbl, "TEMP":dbl})  [unwired: 1 in]
                  }
                }
                "PID-out" <- w2183
              }
              frame #3 {
                n848 = local read "TEMP"() -> (w2222:dbl)
                n849 = Greater Or Equal?(x=w2222, y="Set Temp 2") -> (x >= y?=w2227:bool)
                n850 = case shown="True" w2227 {
                  tunnel: [FALSE TRUE] -> w2225
                  frame False {
                  }
                  frame True {
                  }
                }
                "Status 13" <- w2225
                n851 = And(x=w2225, y="trip1 8") -> (x .and. y?=w2224:bool)
                n852 = case shown="True" w2224 {
                  frame False {
                  }
                  frame True {
                    w2228 = FALSE ("OK Button 2")
                    n853 = local write "Heater Button"(w2228) -> ()
                    n854 = local write "RUN"(w2228) -> ()
                  }
                }
              }
            }
          }
        }
        n855 = stacked-sequence {
          frame #0 {
            n856 = case shown="True" "RST FF" {
              frame False {
              }
              frame True {
                w1968 = 0.0 ("X Scale.Range:Maximum")
                n857 = property on="Frictional Force ( N )" class="WFChart (strict)"("XScale.Maximum"=600.0 ("X Scale.Range:Maximum"), "XScale.Minimum"=w1968, "YScale.Maximum"=10.0 ("Y Scale.Range:Maximum"), "YScale.Minimum"=w1968) -> ()  [unwired: 2 in, 2 out]
              }
            }
          }
          frame #1 {
            n858 = case shown="True" "RST TEMP" {
              frame False {
              }
              frame True {
                n859 = property on="Temperature ( Deg C )" class="WFChart (strict)"("XScale.Minimum"=0.0 ("X Scale.Range:Minimum"), "XScale.Maximum"=600.0 ("X Scale.Range:Maximum"), "YScale.Minimum"=0.0 ("Y Scale.Range:Minimum"), "YScale.Maximum"=100.0 ("Y Scale.Range:Maximum")) -> ()  [unwired: 2 in, 2 out]
              }
            }
          }
          frame #2 {
            n860 = case shown="True" "RSTCOF" {
              frame False {
              }
              frame True {
                n861 = property on="Coefficient of Friction" class="WFChart (strict)"("XScale.Minimum"=0.0 ("X Scale.Range:Minimum"), "XScale.Maximum"=600.0 ("X Scale.Range:Maximum"), "YScale.Maximum"=1.0 ("X Scale.Range:Minimum"), "YScale.Minimum"=0.0 ("X Scale.Range:Minimum")) -> ()  [unwired: 2 in, 2 out]
              }
            }
          }
          frame #3 {
            n862 = case shown="True" "RSTCOF 2" {
              frame False {
              }
              frame True {
                (unwired) 100.0 ("Y Scale.Range:Maximum")
                (unwired) 0.0 ("Y Scale.Range:Minimum")
                (unwired) 600.0 ("X Scale.Range:Maximum")
                (unwired) 0.0 ("X Scale.Range:Minimum")
              }
            }
          }
          frame #4 {
            n863 = case shown="True" "RSTCOF 3" {
              frame False {
              }
              frame True {
                n864 = property on="Electronic contact resistance ( % )" class="WFChart (strict)"("XScale.Minimum"=0.0 ("X Scale.Range:Minimum"), "XScale.Maximum"=600.0 ("X Scale.Range:Maximum"), "YScale.Minimum"=0.0 ("Y Scale.Range:Minimum"), "YScale.Maximum"=100.0 ("Y Scale.Range:Maximum")) -> ()  [unwired: 2 in, 2 out]
              }
            }
          }
        }
        n865 = case shown="True" "Case Constant\n(See Context Help) 13" {
          frame False {
          }
          frame True {
            w1915 = TRUE ("Heater")
            n866 = local write "Humidity"(w1915) -> ()
            n867 = local write "Heater Button"(w1915) -> ()
            n868 = local read "TEST STANDARD"() -> (w1918:T2)
            n869 = local read "TEST STANDARD"() -> (w1913:T2)
            n870 = Equal?(x=w1918, y=enum16{"ASTM D6079", "ISO 12156", "Custom"}."ISO 12156" ("Test Standard")) -> (x = y?=w1916:bool)
            n871 = Equal?(x=w1913, y=enum16{"ASTM D6079", "ISO 12156", "Custom"}."ASTM D6079" ("Test Standard")) -> (x = y?=w1912:bool)
            n872 = case shown="True" w1916 {
              frame False {
              }
              frame True {
                n873 = local write "airtempflg"(FALSE ("airtempflg")) -> ()
                n874 = local write "Heater"(TRUE ("Heater")) -> ()
              }
            }
            n875 = case shown="True" w1912 {
              frame False {
              }
              frame True {
                n876 = local write "airtempflg"(TRUE ("airtempflg")) -> ()
                n877 = local write "Heater"(FALSE ("Heater")) -> ()
              }
            }
          }
        }
        n878 = local read "RUN"() -> (w1859:bool)
        n879 = case shown="True" w1859 {
          tunnel: [FALSE ("TEST RUNNING") TRUE ("TEST RUNNING")] -> w1850
          frame False {
            w1989 = 0.0 ("Flag")
            n880 = local write "Flag"(w1989) -> ()
            n881 = local write "Time Remaining"(w1989) -> ()
            n882 = local write "Elapsed time"(0.0 ("elapsedtime")) -> ()
          }
          frame True {
            n883 = local write "Flag"(10.0 ("Flag")) -> ()
          }
        }
        n884 = local read "Flag"() -> (w1856:dbl)
        n885 = local read "RUN"() -> (w1853:bool)
        n886 = Equal?(x=w1856, y=10.0) -> (x = y?=w1854:bool)
        n887 = Not(x=w1853) -> (.not. x?=w1852:bool)
        n888 = And(x=w1854, y=w1852) -> (x .and. y?=w1851:bool)
        n889 = case shown="True" w1851 {
          frame False {
          }
          frame True {
            w1966 = FALSE ("Heater Button")
            n890 = local write "Heater Button"(w1966) -> ()
            n891 = local write "Humidity"(w1966) -> ()
          }
        }
        n892 = local write "Save"(w1850) -> ()
        n893 = local write "Test \nStatus"(w1850) -> ()
        n894 = local write "st enable"(w1850) -> ()
        n895 = local write "PWR"(w1850) -> ()
        n896 = local read "Set Temp"() -> (w1812:dbl)
        n897 = local read "SetTemp"() -> (w1814:dbl)
        n898 = local read "Set Rh"() -> (w1813:dbl)
        n899 = local read "Amb temp"() -> (w1811:dbl)
        n900 = local read "Humidity ( Rh )"() -> (w1810:dbl)
        n901 = local read "TEMP"() -> (w1809:dbl)
        n902 = Add(x=w1814, y=w1839) -> (x+y=w1840:dbl)
        n903 = Subtract(x=w1814, y=w1839) -> (x-y=w1841:dbl)
        n904 = Add(x=w1813, y=w1838) -> (x+y=w1837:dbl)
        n905 = Subtract(x=w1813, y=w1838) -> (x-y=w1836:dbl)
        n906 = Add(x=w1812, y=w1833) -> (x+y=w1834:dbl)
        n907 = Subtract(x=w1812, y=w1833) -> (x-y=w1835:dbl)
        n908 = In Range and Coerce(upper limit=w1840, x=w1811, lower limit=w1841) -> (In Range?=w1830:bool)  [unwired: 1 out]
        n909 = In Range and Coerce(upper limit=w1837, x=w1810, lower limit=w1836) -> (In Range?=w1828:bool)  [unwired: 1 out]
        n910 = In Range and Coerce(upper limit=w1834, x=w1809, lower limit=w1835) -> (In Range?=w1826:bool)  [unwired: 1 out]
        n911 = case shown="True" w1830 {
          tunnel: [FALSE ("RUN") TRUE ("RUN")] -> w1829
          tunnel: [_ 1] -> w1822
          frame False {
          }
          frame True {
          }
        }
        n912 = case shown="True" w1828 {
          tunnel: [FALSE ("RUN") TRUE ("RUN")] -> w1827
          tunnel: [_ 2] -> w1821
          frame False {
          }
          frame True {
          }
        }
        n913 = case shown="True" w1826 {
          tunnel: [FALSE ("RUN") TRUE ("RUN")] -> w1825
          tunnel: [_ 3] -> w1820
          frame False {
          }
          frame True {
          }
        }
        n914 = local read "airtempflg"() -> (w1831:bool)
        n915 = Or(x=w1831, y=w1829) -> (x .or. y?=w1832:bool)
        n916 = Build Array(w1822, w1821, w1820) -> (w1818:i32[])
        n917 = Compound Arithmetic op=AND(w1832, w1827, w1825) -> ()  [unwired: 1 out]
        n918 = case shown="True" "Case Constant\n(See Context Help) 14" {
          frame False {
          }
          frame True {
            w1909 = FALSE ("autostrtflg")
            n919 = local write "autostrtflg"(w1909) -> ()
            n920 = local write "autostart"(w1909) -> ()
            n921 = local write "RUN"(TRUE ("RUN")) -> ()
            n922 = local write "String 14"(" Running....." ("String 14")) -> ()
          }
        }
        n923 = Insert Into Array(array=string[] ["Air Temperature has reached set value,", "Humidity has reached set value,", "Sample Temperaturehas reached set value,", ""], index=0, new element="") -> (w1817:string[])
        n924 = for {
          tunnel: w1818 -> [w1899] mode=indexing
          tunnel: w1817 -> [w1898]
          shift-right: [w1895] -> w1816
          shift-left: "" -> [w1897]
          n925 = Index Array(array=w1898, index=w1899) -> (element=w1896:string)
          n926 = Concatenate Strings(w1896, w1897) -> (w1895:string)
        }
        n927 = local write "autostart 2"(w1816) -> ()
      }
      frame 1 {
        # "Elapsed time\ncof\nstroke\nAir temp\nTemp\nHumidity"
        n928 = case shown="True" "OPEN 4" {
          frame False {
          }
          frame True {
            (unwired) 0  # existing file
            w2419 = "Choose a datalog file to open"  # prompt
            n929 = local write "OPEN 4"(FALSE ("OPEN 1")) -> ()
            n930 = String To Path(string="C:\\LAB-IQ-NXT\\Data\\") -> (path=w2404:path)
            n931 = File Dialog(6:"*.dgf" ("pattern"), 7:w2419, 11:w2404) -> (0:w2402:errorcluster, 3:w2410:path)  [unwired: 4 in, 2 out]
            n932 = Unbundle(w2402) -> ()  [unwired: 3 out]
            n933 = Path To String(path=w2410) -> (string=w2405:string)
            "string1 4" <- w2405
            n934 = Match Pattern(string=w2405, regular expression=".dgf" ("substring (\"\")")) -> (before substring=w2415:string)  [unwired: 1 in, 3 out]
            n935 = Concatenate Strings(w2415, ".duf" ("Substring")) -> (w2412:string)
            n936 = String To Path(string=w2412) -> (path=w2416:path)
            n937 = call <vilib>:"Read Characters From File.vi"("file path (dialog if empty)"=w2416, "start of read offset (chars.:0)"=60 ("start of read offset (chars.: 0)")) -> ("character string"=→"String Control 8":string)  [unwired: 4 in, 3 out]
            n938 = Strip Path(path=w2410) -> (name=w2408:string)  [unwired: 1 out]
            n939 = Match Pattern(string=w2408, regular expression=".dgf") -> (before substring=→"String Control 7":string)  [unwired: 1 in, 3 out]
          }
        }
        n940 = case shown="True" "OPEN 3" {
          frame False {
          }
          frame True {
            (unwired) 0  # existing file
            w2401 = "Choose a datalog file to open"  # prompt
            n941 = local write "OPEN 3"(FALSE ("OPEN 1")) -> ()
            n942 = String To Path(string="C:\\LAB-IQ-NXT\\Data\\") -> (path=w2386:path)
            n943 = File Dialog(6:"*.dgf" ("pattern"), 7:w2401, 11:w2386) -> (0:w2384:errorcluster, 3:w2392:path)  [unwired: 4 in, 2 out]
            n944 = Unbundle(w2384) -> ()  [unwired: 3 out]
            n945 = Path To String(path=w2392) -> (string=w2387:string)
            "string1 3" <- w2387
            n946 = Match Pattern(string=w2387, regular expression=".dgf" ("substring (\"\")")) -> (before substring=w2397:string)  [unwired: 1 in, 3 out]
            n947 = Concatenate Strings(w2397, ".duf" ("Substring")) -> (w2394:string)
            n948 = String To Path(string=w2394) -> (path=w2398:path)
            n949 = call <vilib>:"Read Characters From File.vi"("file path (dialog if empty)"=w2398, "start of read offset (chars.:0)"=60 ("start of read offset (chars.: 0)")) -> ("character string"=→"String Control 6":string)  [unwired: 4 in, 3 out]
            n950 = Strip Path(path=w2392) -> (name=w2390:string)  [unwired: 1 out]
            n951 = Match Pattern(string=w2390, regular expression=".dgf") -> (before substring=→"String Control 5":string)  [unwired: 1 in, 3 out]
          }
        }
        n952 = case shown="True" "OPEN 2" {
          frame False {
          }
          frame True {
            (unwired) 0  # existing file
            w2383 = "Choose a datalog file to open"  # prompt
            n953 = local write "OPEN 2"(FALSE ("OPEN 1")) -> ()
            n954 = String To Path(string="C:\\LAB-IQ-NXT\\Data\\") -> (path=w2368:path)
            n955 = File Dialog(6:"*.dgf" ("pattern"), 7:w2383, 11:w2368) -> (0:w2366:errorcluster, 3:w2374:path)  [unwired: 4 in, 2 out]
            n956 = Unbundle(w2366) -> ()  [unwired: 3 out]
            n957 = Path To String(path=w2374) -> (string=w2369:string)
            "string1 2" <- w2369
            n958 = Match Pattern(string=w2369, regular expression=".dgf" ("substring (\"\")")) -> (before substring=w2380:string)  [unwired: 1 in, 3 out]
            n959 = Concatenate Strings(w2380, ".duf" ("Substring")) -> (w2377:string)
            n960 = String To Path(string=w2377) -> (path=w2375:path)
            n961 = call <vilib>:"Read Characters From File.vi"("file path (dialog if empty)"=w2375, "start of read offset (chars.:0)"=60 ("start of read offset (chars.: 0)")) -> ("character string"=→"String Control 4":string)  [unwired: 4 in, 3 out]
            n962 = Strip Path(path=w2374) -> (name=w2372:string)  [unwired: 1 out]
            n963 = Match Pattern(string=w2372, regular expression=".dgf") -> (before substring=→"String Control 3":string)  [unwired: 1 in, 3 out]
          }
        }
        n964 = case shown="True" "OPEN 1" {
          frame False {
          }
          frame True {
            (unwired) 0  # existing file
            w2365 = "Choose a datalog file to open"  # prompt
            n965 = local write "OPEN 1"(FALSE ("OPEN 1")) -> ()
            n966 = String To Path(string="C:\\LAB-IQ-NXT\\Data\\") -> (path=w2350:path)
            n967 = File Dialog(6:"*.dgf" ("pattern"), 7:w2365, 11:w2350) -> (0:w2348:errorcluster, 3:w2356:path)  [unwired: 4 in, 2 out]
            n968 = Unbundle(w2348) -> ()  [unwired: 3 out]
            n969 = Path To String(path=w2356) -> (string=w2351:string)
            "string1" <- w2351
            n970 = Match Pattern(string=w2351, regular expression=".dgf" ("substring (\"\")")) -> (before substring=w2361:string)  [unwired: 1 in, 3 out]
            n971 = Concatenate Strings(w2361, ".duf" ("Substring")) -> (w2357:string)
            n972 = String To Path(string=w2357) -> (path=w2362:path)
            n973 = call <vilib>:"Read Characters From File.vi"("file path (dialog if empty)"=w2362, "start of read offset (chars.:0)"=60 ("start of read offset (chars.: 0)")) -> ("character string"=→"String Control 2":string)  [unwired: 4 in, 3 out]
            n974 = Strip Path(path=w2356) -> (name=w2355:string)  [unwired: 1 out]
            n975 = Match Pattern(string=w2355, regular expression=".dgf") -> (before substring=→"String Control":string)  [unwired: 1 in, 3 out]
          }
        }
        n976 = case shown="True" "RSTV1 4" {
          frame False {
          }
          frame True {
            n977 = property on="Stroke" class="XYGraph (strict)"("Y Scale.Display Format:Precision"=u8 2 ("Y Scale.Format & Precision:Precision")) -> ()  [unwired: 2 in, 2 out]
            n978 = property on="Stroke" class="XYGraph (strict)"("X Scale.Range:Minimum"=0.0 ("Y Scale.Range:Maximum"), "X Scale.Range:Maximum"=75.0 ("X Scale.Range:Minimum"), "Y Scale.Range:Minimum"=0.98, "Y Scale.Range:Maximum"=1.02) -> ()  [unwired: 2 in, 2 out]
          }
        }
        n979 = case shown="True" "rstv2" {
          frame False {
          }
          frame True {
            n980 = property on="Coefficient Of Friction" class="XYGraph (strict)"("X Scale.Range:Minimum"=0.0 ("Y Scale.Range:Maximum"), "X Scale.Range:Maximum"=75.0, "Y Scale.Range:Minimum"=0.0, "Y Scale.Range:Maximum"=1.0 ("X Scale.Range:Minimum")) -> ()  [unwired: 2 in, 2 out]
            n981 = property on="Coefficient Of Friction" class="XYGraph (strict)"("Y Scale.Display Format:Precision"=u8 3 ("Y Scale.Format & Precision:Precision")) -> ()  [unwired: 2 in, 2 out]
          }
        }
        n982 = case shown="True" "RSTV1 3" {
          frame False {
          }
          frame True {
            n983 = property on="Air Temperature" class="XYGraph (strict)"("X Scale.Range:Minimum"=0.0 ("Y Scale.Range:Minimum"), "X Scale.Range:Maximum"=75.0 ("Y Scale.Range:Maximum"), "Y Scale.Range:Minimum"=20.0 ("X Scale.Range:Minimum"), "Y Scale.Range:Maximum"=26.0 ("X Scale.Range:Maximum")) -> ()  [unwired: 2 in, 2 out]
            n984 = property on="Air Temperature" class="XYGraph (strict)"("Y Scale.Display Format:Precision"=u8 2 ("Y Scale.Format & Precision:Precision")) -> ()  [unwired: 2 in, 2 out]
          }
        }
        n985 = case shown="True" "RST CP" {
          frame False {
          }
          frame True {
            n986 = property on="Sample Temperature" class="XYGraph (strict)"("X Scale.Range:Minimum"=0.0, "X Scale.Range:Maximum"=75.0, "Y Scale.Range:Minimum"=58.0, "Y Scale.Range:Maximum"=62.0) -> ()  [unwired: 2 in, 2 out]
            n987 = property on="Sample Temperature" class="XYGraph (strict)"("Y Scale.Display Format:Precision"=u8 2 ("Y Scale.Format & Precision:Precision")) -> ()  [unwired: 2 in, 2 out]
          }
        }
        n988 = case shown="True" "RST CP 2" {
          frame False {
          }
          frame True {
            n989 = property on="XY Graph 13" class="XYGraph (strict)"("X Scale.Range:Minimum"=0.0, "X Scale.Range:Maximum"=75.0, "Y Scale.Range:Minimum"=0.0, "Y Scale.Range:Maximum"=100.0) -> ()  [unwired: 2 in, 2 out]
            n990 = property on="XY Graph 13" class="XYGraph (strict)"("Y Scale.Display Format:Precision"=u8 0 ("Y Scale.Format & Precision:Precision")) -> ()  [unwired: 2 in, 2 out]
          }
        }
        n991 = case shown="True" "RSTV1 2" {
          frame False {
          }
          frame True {
            n992 = property on="Humidity" class="XYGraph (strict)"("X Scale.Range:Minimum"=0.0, "X Scale.Range:Maximum"=75.0, "Y Scale.Range:Minimum"=48.0, "Y Scale.Range:Maximum"=58.0) -> ()  [unwired: 2 in, 2 out]
            n993 = property on="Humidity" class="XYGraph (strict)"("Y Scale.Display Format:Precision"=u8 0 ("Y Scale.Format & Precision:Precision")) -> ()  [unwired: 2 in, 2 out]
          }
        }
        n994 = case shown="True" "RST CP 3" {
          frame False {
          }
          frame True {
            n995 = property on="Air Temp vs Rh" class="XYGraph (strict)"("X Scale.Range:Minimum"=18.0, "X Scale.Range:Maximum"=28.0 ("X Scale.Range:Minimum"), "Y Scale.Range:Minimum"=30.0 ("X Scale.Range:Minimum"), "Y Scale.Range:Maximum"=70.0 ("X Scale.Range:Minimum")) -> ()  [unwired: 2 in, 2 out]
          }
        }
      }
      frame 2 {
        # "Elapsed time\ncof\nstroke\nmean pos\nTemp\nHumidity"
        n996 = case shown="True" "Export" {
          frame False {
          }
          frame True {
            w2550 = "                                      " ("string")
            w2552 = "\r"
            (unwired) i16 6 ("width (-)")
            w2629 = "\r"
            w2561 = "\r"
